vi "Nufi Dryer Debug Message Buff.vi"(10 "New String":string, 11 "Partial Message String":string) -> (1 "Partial Message FWD":string, 2 "Full Message to Save":string, 3 "Message to Save":bool, 4 "Number of Messages":i32, 5 "More Full Messages?":bool)   [LabVIEW 2016]
uses:
  <vilib>/Utility/error.llb/whitespace.ctl
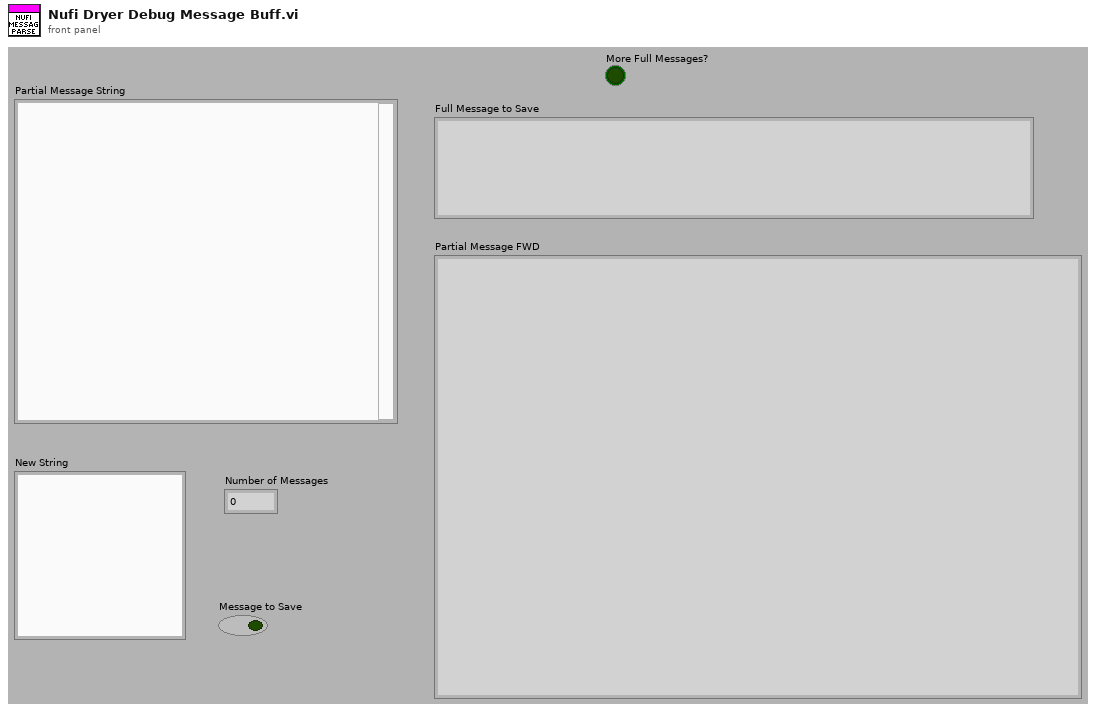
[diagram p1: front panel]
types:
  T1 = typedef "whitespace.ctl" = u16
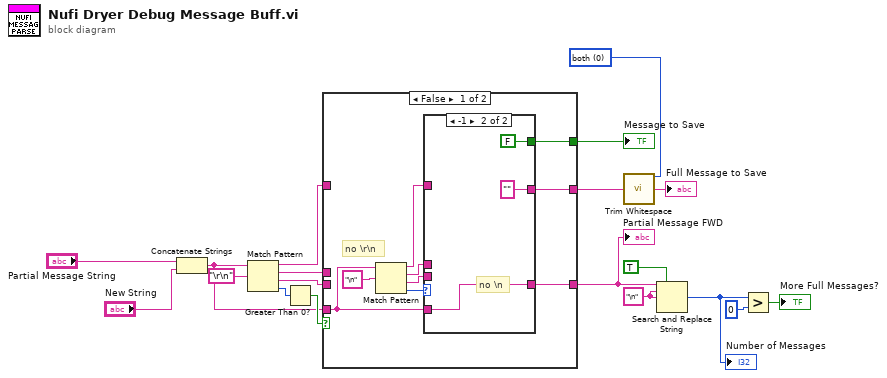
[diagram p0: block diagram]
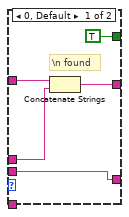
[diagram p2: hidden frame]
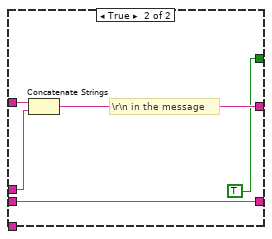
[diagram p3: hidden frame]
diagram:
  w1 = T1 0 items=["both", "start of string", "end of string"] ("location (both)")
  w7 = "\n" ("regular expression")
  n1 = Concatenate Strings("Partial Message String", "New String") -> (w11:string)
  n2 = Match Pattern(string=w11, regular expression="\r\n") -> (before substring=w13:string, match substring=w12:string, after substring=w14:string, offset past match=w17:i32)  [unwired: 1 in]
  n3 = Greater Than 0?(x=w17) -> (x > 0?=w15:bool)
  n4 = case shown="False" w15 {
    tunnel: [w23 w41] -> w9
    tunnel: w14 -> [_ w41]
    tunnel: w13 -> [_ w40]
    tunnel: w12 -> [_ w39]
    tunnel: [w24 w38] -> w3
    tunnel: w11 -> [w21 _]
    tunnel: [w26 TRUE ("Message to Save")] -> w10
    frame False {
      # "no \\r\\n"
      n5 = Match Pattern(string=w21, regular expression="\n") -> (before substring=w25:string, match substring=w20:string, after substring=w22:string, offset past match=w27:i32)  [unwired: 1 in]
      n6 = case shown="-1" w27 {
        tunnel: [TRUE ("Message to Save") FALSE ("Message to Save")] -> w26
        tunnel: w25 -> [w31 _]
        tunnel: [w29 ""] -> w24
        tunnel: [w32 w35] -> w23
        tunnel: w22 -> [w32 _]
        tunnel: w21 -> [_ w35]
        tunnel: w20 -> [w30 _]
        frame 0, Default {
          # "\\n found"
          n7 = Concatenate Strings(w31, w30) -> (w29:string)
        }
        frame -1 {
          # "no \\n"
        }
      }
    }
    frame True {
      # "\\r\\n in the message"
      n8 = Concatenate Strings(w40, w39) -> (w38:string)
    }
  }
  "Partial Message FWD" <- w9
  "Message to Save" <- w10
  n9 = call <vilib>:"Trim Whitespace.vi"("string"=w3, "location (both)"=w1) -> ("trimmed string"=→"Full Message to Save":string)
  n10 = Search and Replace String(replace all?=TRUE ("replace all? (F)"), input string=w9, search string=w7, replace string=w7) -> (number of replacements=w6:i32)  [unwired: 4 in, 3 out]
  "Number of Messages" <- w6
  n11 = Greater?(x=w6, y=0) -> (0:→"More Full Messages?":bool)
